vi "NI 5772 (AC) - Digitizer_vDirectDataSend (FPGA).vi"() -> ()   [LabVIEW 2020]
doc: "Example Description:\nThis example demonstrates how to enable Time Interleaved Sampling with the NI 5772 adapter module to achieve a sampling rate of 1.6GS/s. This example continuously acquires records of analog input data from the NI 5772 adapter module. It allows you to select an AI channel, trigger type, and record size. This VI must be compiled before it is run. \n\nRunning the VI:\nThis VI must be run from the NI 5772 - Getting Started (Host).vi. Refer to the host VI documentation for steps regarding running and configuring the FPGA VI. \n\nExecution Steps:\nRefer to the Block Diagram of this VI for execution comments."
uses:
  Controls/AI Trigger Type.ctl
  Controls/Aquire State.ctl
  <vilib>/Platform/TimedLoop/XDataNode/timing_clust.ctl
  <vilib>/Platform/TimedLoop/XDataNode/nitl_modes.ctl
  <vilib>/Platform/TimedLoop/XDataNode/wakeup.ctl
  <vilib>/rvi/Emulation/niFpgaGetClockAttributes.vi
  <vilib>/rvi/Emulation/niFpgaSctlEmulationGetInTimedLoop.vi
  <vilib>/rvi/Emulation/niFpgaEmulationReportErrorSimple.vi
  <vilib>/rvi/eio/common/nirviEmuTemplateMethod_errors.vi
  <vilib>/rvi/Emulation/niFpgaCriticalErrorInLSC.vi
  <vilib>/rvi/Emulation/niFpgaProcessEmulError.vi
  <vilib>/rvi/Emulation/niFpgaEmulationIsFPGAContextNoSignature.vi
  <vilib>/rvi/errors/niFpgaSetErrorForExecOnDevCompSimple.vi
  <vilib>/rvi/eio/common/nirviEmuReportErrorAndStop.vi
  <vilib>/rvi/DataTransferAndStorage/Container/Common/niFpgaContainerGetUniqueNameForEmu.vi
  <vilib>/rvi/FIFO/Fifo_Resource/nirvififoEmulationSetSize.vi
  <vilib>/rvi/FIFO/Fifo_Resource/nirviFifoEmulationQueueMgr.vi
  <instcachedir>/0/nirviFifoEmulationQueueMgr_E5CAEC123FF24DC58D834DCA3CDAA9B5.lvgen/nirviFifoEmulationQueueMgr_E5CAEC123FF24DC58D834DCA3CDAA9B5_004.vi
  <vilib>/Utility/error.llb/Clear Errors.vi
  <vilib>/rvi/FIFO/Fifo_Resource/nirvififoEmulationCreateLock.vi
  <vilib>/rvi/FIFO/Fifo_Resource/nirvififoEmulationObtainLock.vi
  <vilib>/rvi/FIFO/Fifo_Resource/nirvififoEmulationReleaseLock.vi
  <vilib>/rvi/occurrence/nirviWaitOnOccurrenceBase.vi
  <vilib>/rvi/errors/nirviReportUnexpectedCaseInternalError.vi
  <vilib>/rvi/errors/nirviReportUnexpectedCaseInternalError (U32).vi
  <instcachedir>/0/nirviFifoEmulationQueueMgr_E5CAEC123FF24DC58D834DCA3CDAA9B5.lvgen/nirviFifoEmulationQueueMgr_E5CAEC123FF24DC58D834DCA3CDAA9B5_000.vi
  <vilib>/rvi/interface/RandomDataEmulation/niFpgaRandomDataHandleErrors.vi
  <vilib>/rvi/FIFO/Fifo_Resource/nirvififoEmulationDetermineInputValidOut.vi
  <instrlib>/_niInstr/Basic Elements/v1/FPGA/Private/Count Up U64.vi
  <vilib>/eio/EIONode/EIONode.xnode
  <vilib>/rvi/DataTransferAndStorage/Container/XNode/niFpgaContainer.xnode
  <vilib>/rvi/FIFO/Fifo_Resource/nirvififoEmulationRead.vi
  <vilib>/Platform/TimedLoop/XDataNode/XDataNode.xnode
  <vilib>/rvi/interface/RandomDataEmulation/nirviRandomDataFpgaReadWriteTemplate.vi
  <vilib>/rvi/FIFO/Fifo_Resource/nirvififoEmulationWrite.vi
  <vilib>/Platform/TimedLoop/XDataNode/XDNodeRunTimeDep.lvlib
  <instrlib>/_niInstr/Basic Elements/v1/FPGA/niInstr Basic Elements v1 FPGA.lvlib
  Controls/DigitizerState.ctl
  <vilib>/rvi/FIFO/Fifo_Resource/nirvififoEmulationGetNumberOfElementsToRead.vi
  <vilib>/rvi/Memory/Memory_Emulation/nirvimemoryFastEmulation.vi
  <vilib>/rvi/Memory/Memory_Emulation/nirvimemoryEmulation.vi
panel:
  out "DMA FIFO Overflow? 3":bool caption="FIFO Overflow?"
  out "DMA FIFO Overflow? 2":bool caption="FIFO Overflow?"
  out "WaitForWave\nCompletion":u16
  in  "Wave Sampling Rate":sgl
  in  "WaveSampleCount":sgl format="%#_13g"
  in  "Delay (us)":sgl
  in  "AvgCount_powerOf2":i16=1
  out "DMA FIFO Overflow?":bool caption="FIFO Overflow?"
  out "Removed\nElement":u64
  out "AvgCount":u16=1
  in  "vi/nGenTrig":bool
  in  "TrigIn Simulate":bool
  out "Trig Count":u64
  in  "Clear Count":bool
  out "Delay after Trig [cycles]":u16
  out "TS FIFO In Overflow?":bool caption="FIFO Overflow?"
  in  "Samples Per Trigger":u16=512 min=1 step=1
  in  "Arm Trigger":bool
  in  "User Command Commit":bool
  in  "User Command":u8
  out "User Command Idle":bool
  out "User Command Status":u8
  in  "User Data 0":u16
  in  "User Data 1":u8
  out "PLL Locked":bool
  out "User Error":bool
  out "Configured?":bool
  in  "Trigger Level":i16
  in  "Trigger Type":T1
  # "Resource Configuration"
  # "Analog Input"
  # "Clock Configuration"
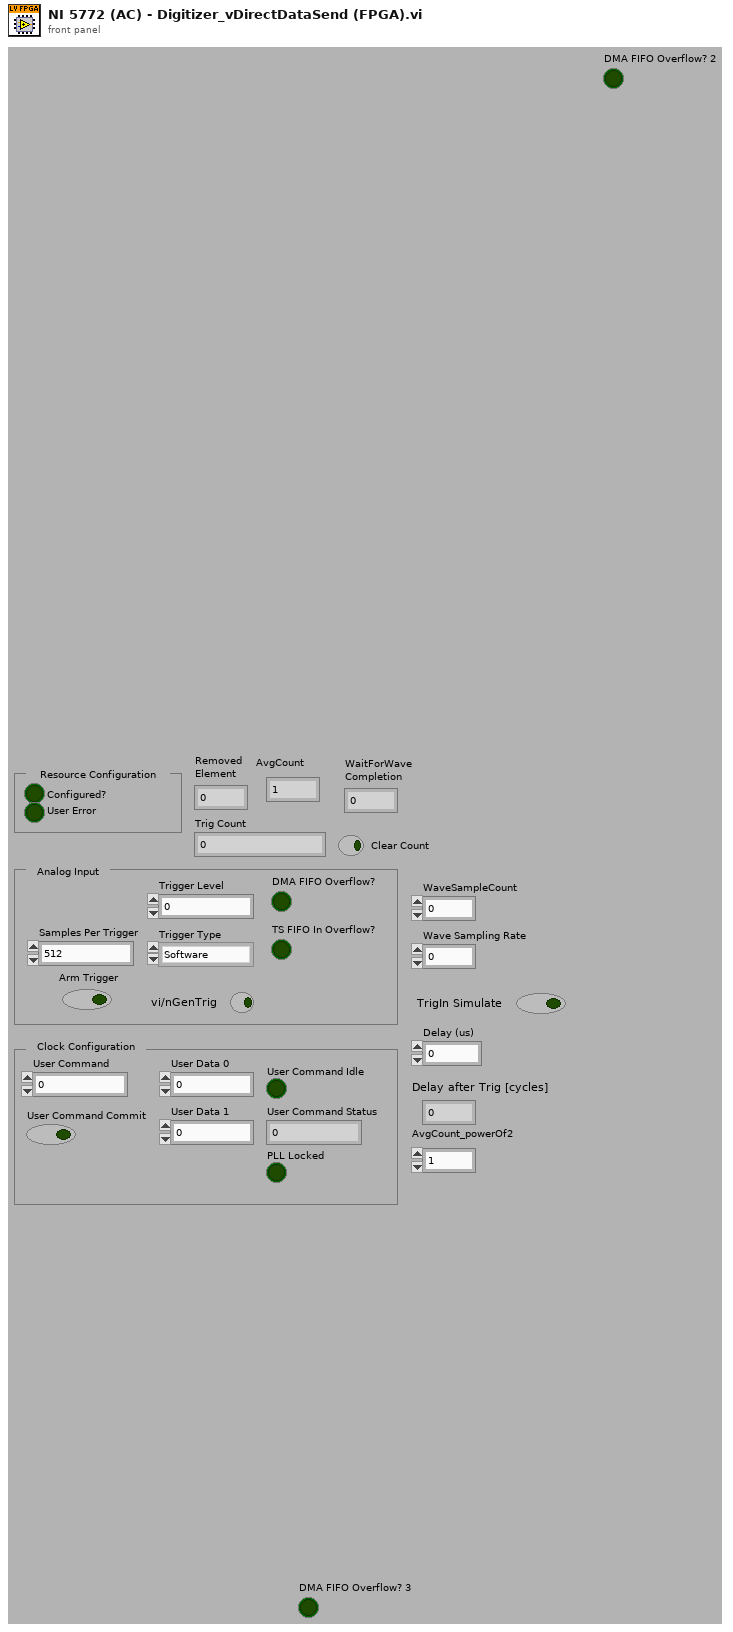
[diagram p1: front panel]
types:
  T1 = typedef "AI Trigger Type.ctl" = enum8{"Software", "Data Edge"}
  T2 = typedef "Aquire State.ctl" = enum8{"Idle", "Wait for Trigger", "AlignWave", "Hold Aquire", "Acquire", "WaitForWaveCompletion", "CheckAvg"}
  T3 = typedef "DigitizerState.ctl" = enum16{"Init", "Build/Clear Accumulator", "GetData", "AverageCountCheck", "SendtoHost"}
  T4 = typedef "XDNodeRunTimeDep.lvlib/timing_clust.ctl" = cluster{"Expected End [f-1]":u64, "Actual End [f-1]":u64, "Finished Late? [f-1]":bool, "Expected End [i-1]":u64, "Actual End [i-1]":u64, "Finished Late? [i-1]":bool, "Expected Start [i]":u64, "Actual Start [i]":u64, "Expected Start [f]":u64, "Actual Start [f]":u64, "Source Name":string, "Structure Name":string, "Period":i64, "Deadline":i64, "Offset":i64, "Start":i64, "Priority":i32, "Timeout":i32, "Mode":T5, "Wakeup Reason":T6, "Error":errorcluster, "Source Type":string, "Secondary Source Type":string, "Global End Time":u64, "Global Start Time":u64, "Frame Duration":u64, "Iteration Duration":u64, "Assigned CPU":i32, "I/O Scan Engine Mode":u32}
  T5 = typedef "XDNodeRunTimeDep.lvlib/nitl_modes.ctl" = enum32{"No Change", "Process missed periods, maintain original phase", "Discard missed periods, maintain original phase", "Process missed periods, ignore original phase", "Discard missed periods, ignore original phase"}
  T6 = typedef "XDNodeRunTimeDep.lvlib/wakeup.ctl" = enum32{"Normal", "Aborted", "Asynchronous wakeup", "Timing source error", "Timed loop error", "Timeout"}
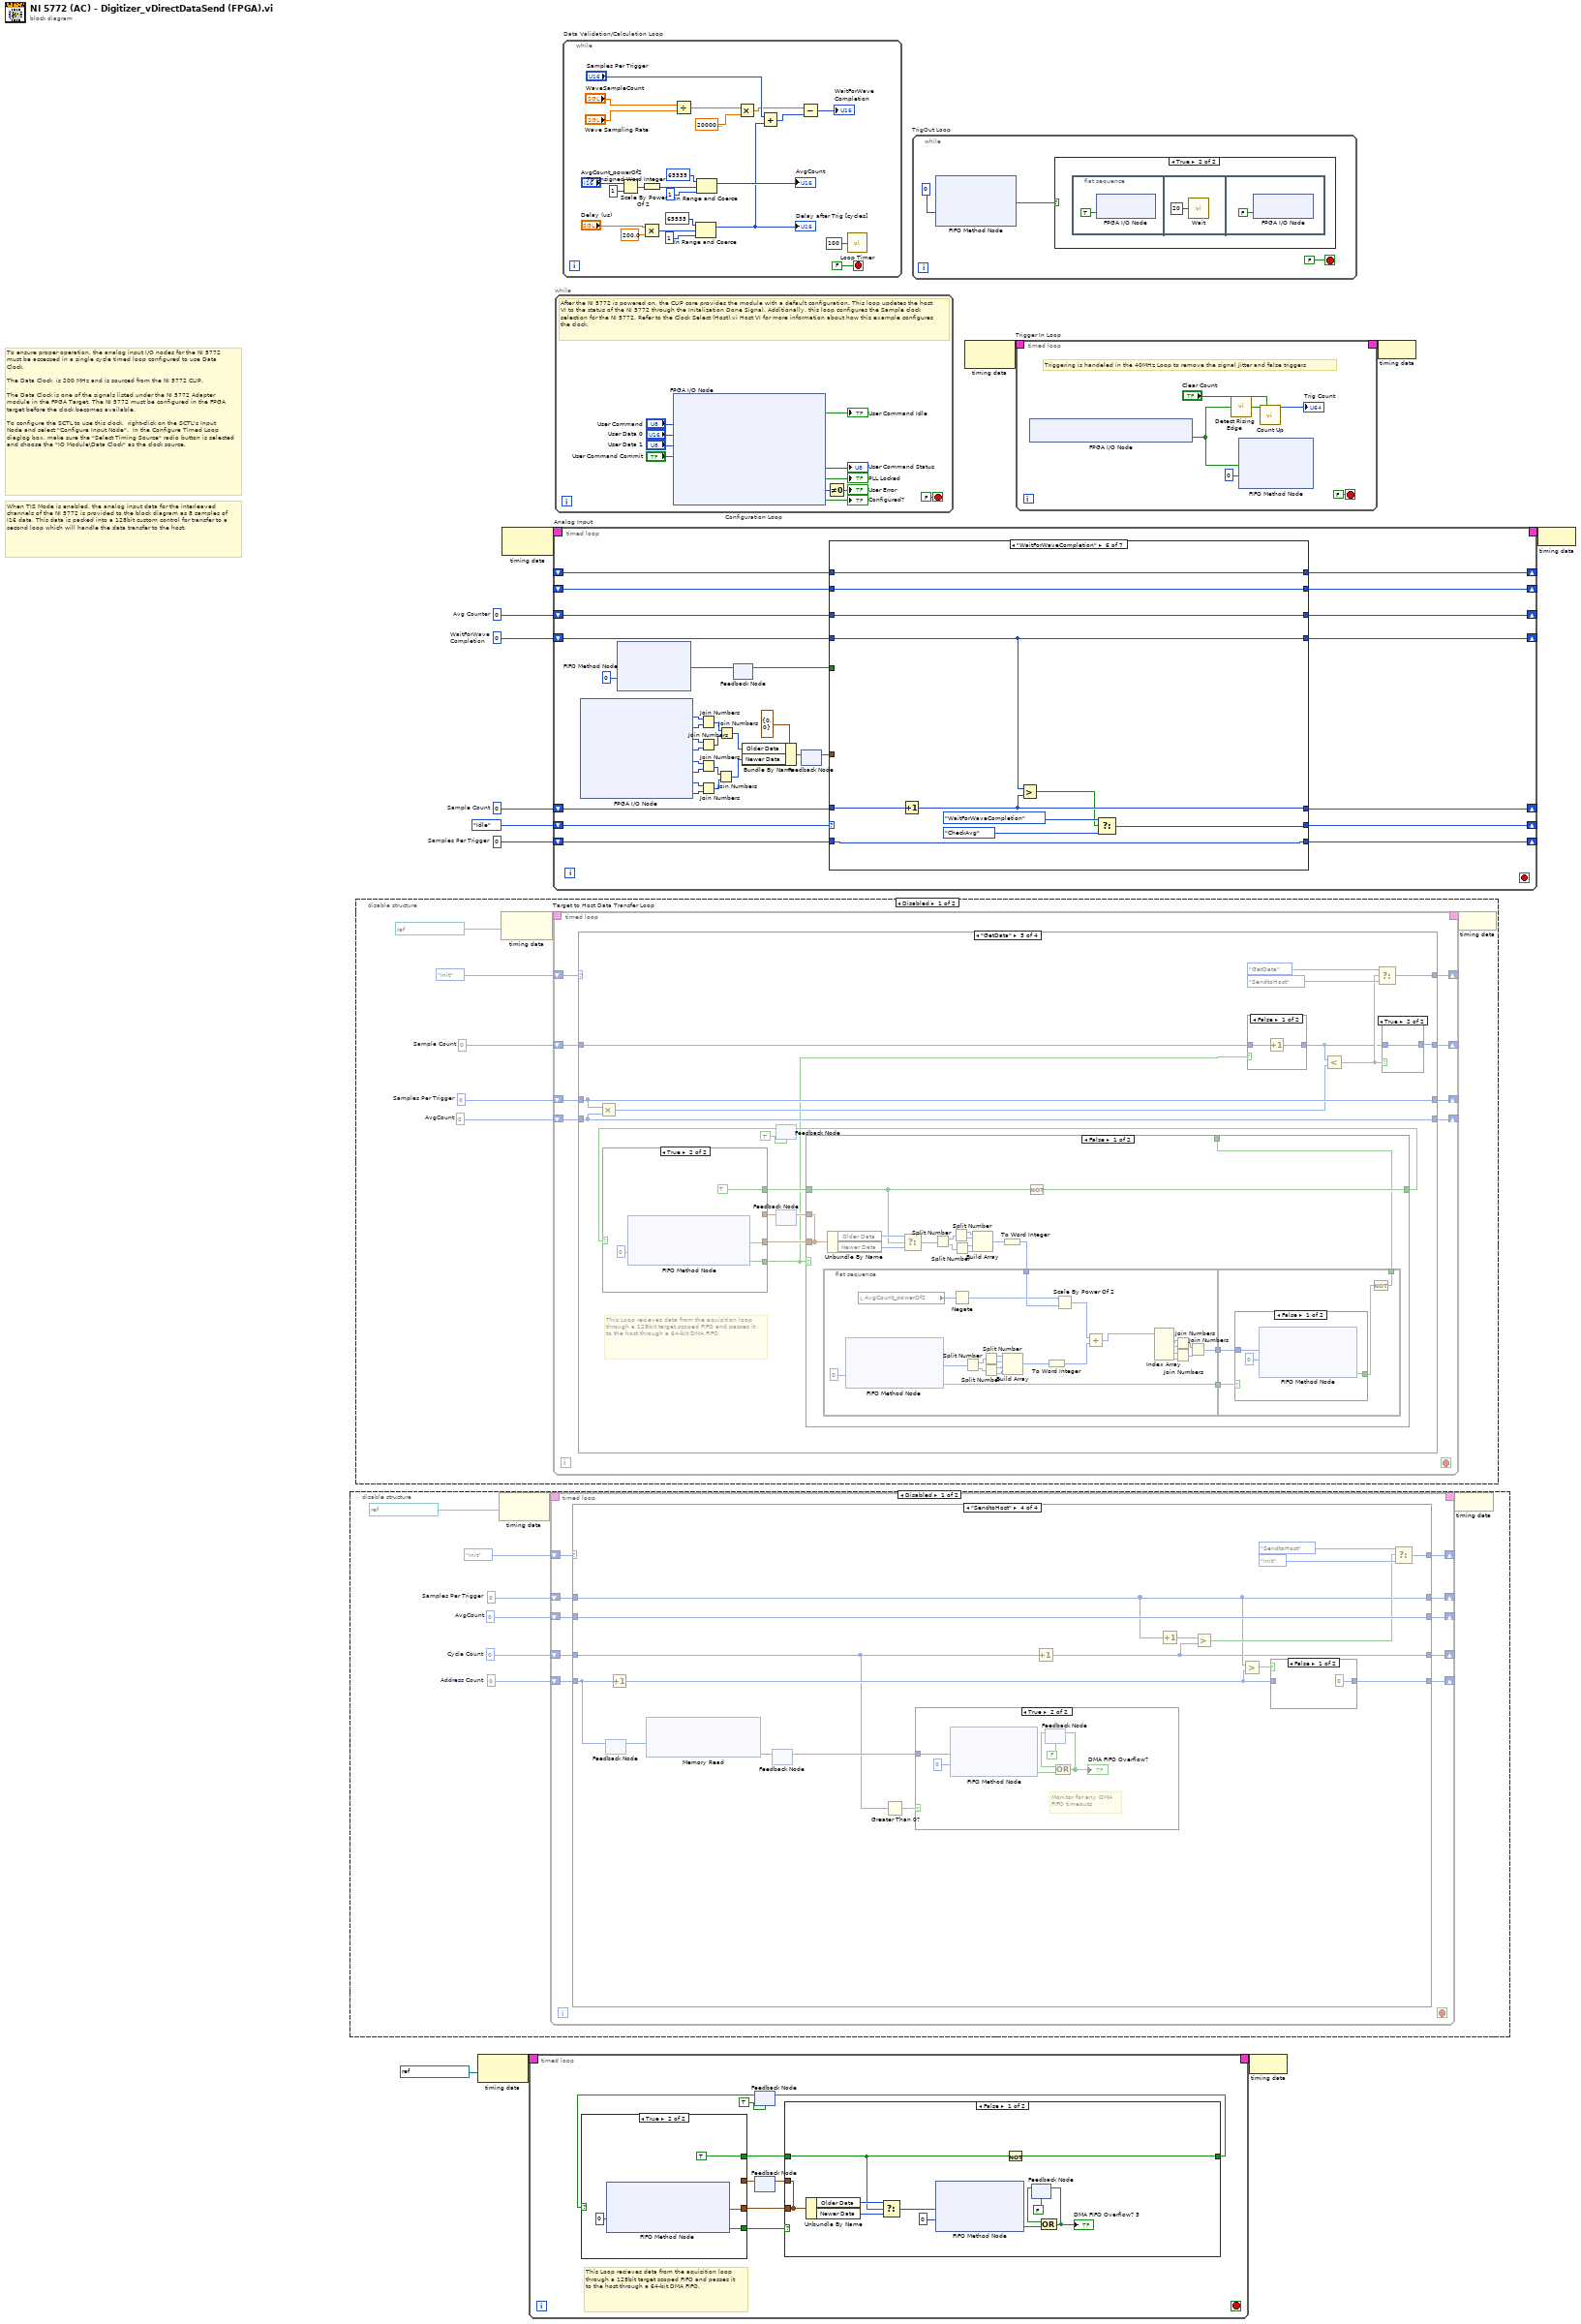
[diagram p0: block diagram]
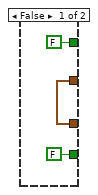
[diagram p2: hidden frame]
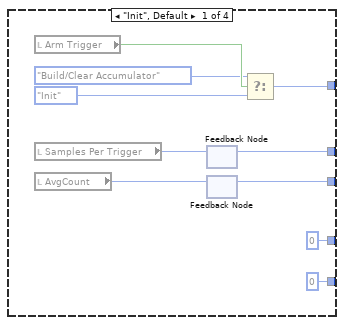
[diagram p4: hidden frame]
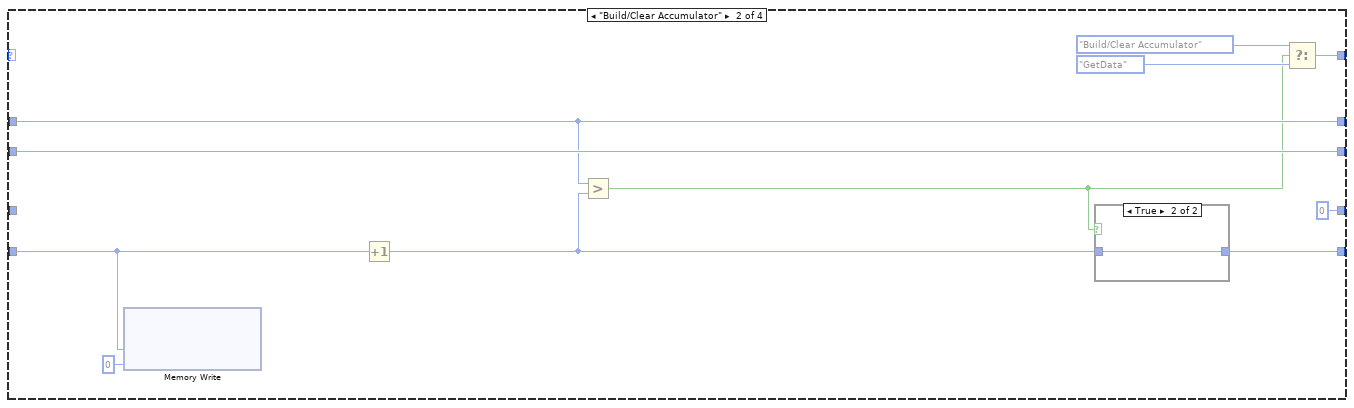
[diagram p5: hidden frame]
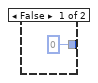
[diagram p6: hidden frame]
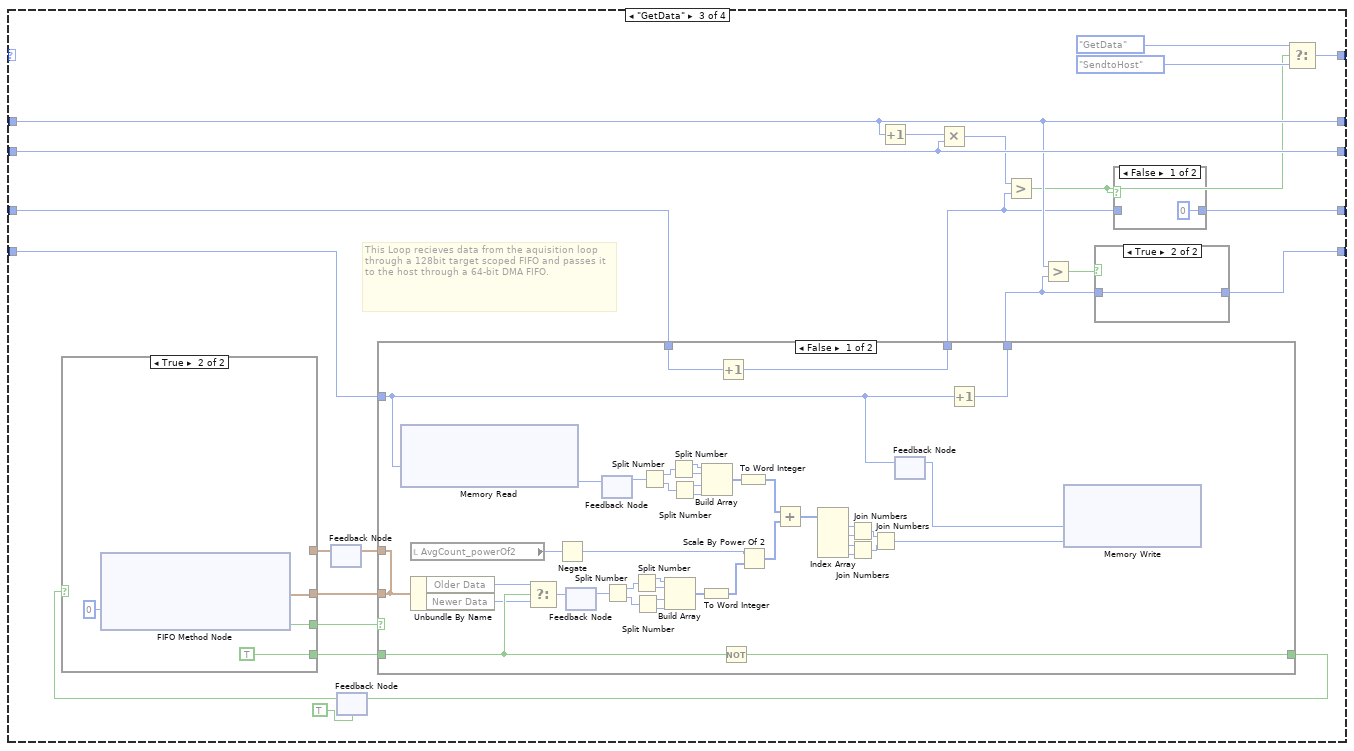
[diagram p7: hidden frame]
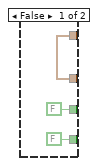
[diagram p9: hidden frame]
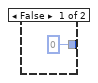
[diagram p11: hidden frame]
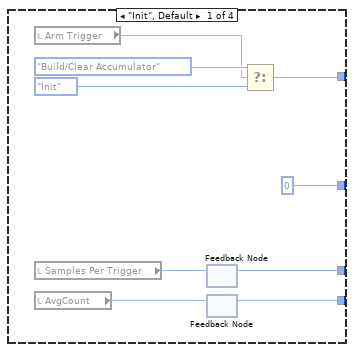
[diagram p15: hidden frame]
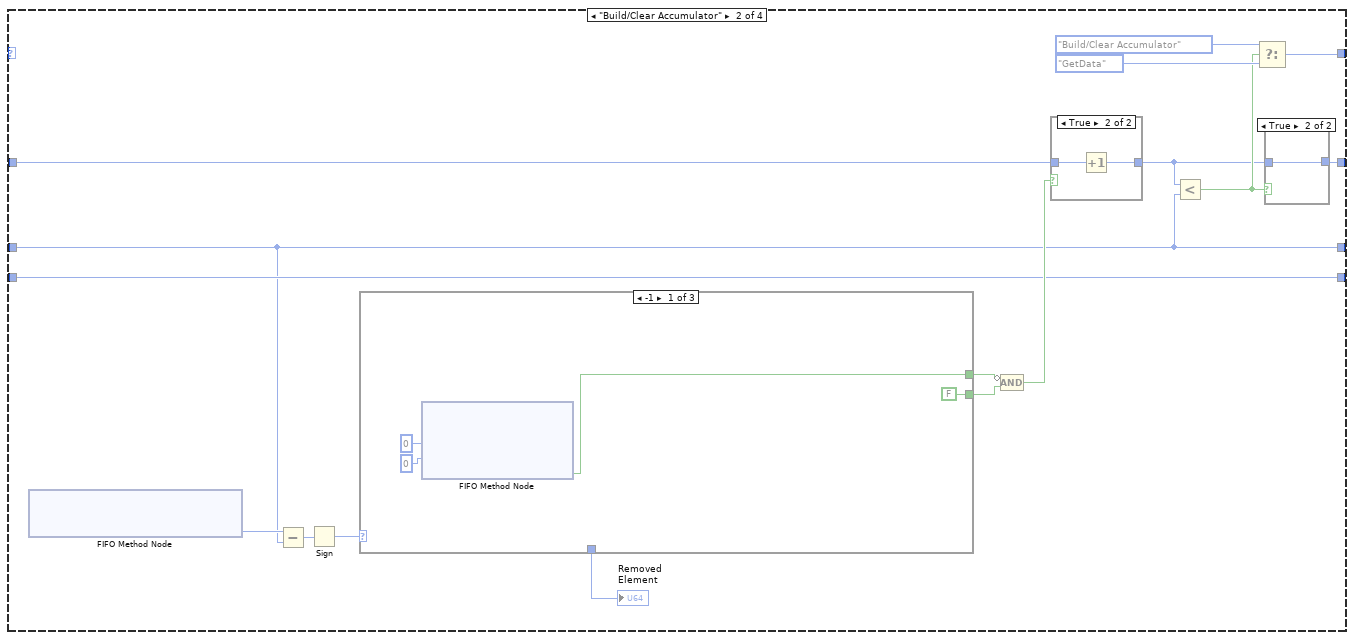
[diagram p16: hidden frame]
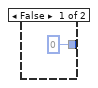
[diagram p17: hidden frame]
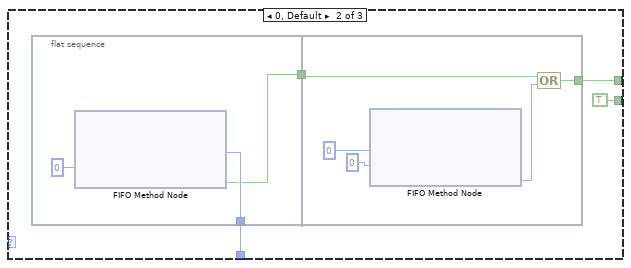
[diagram p19: hidden frame]
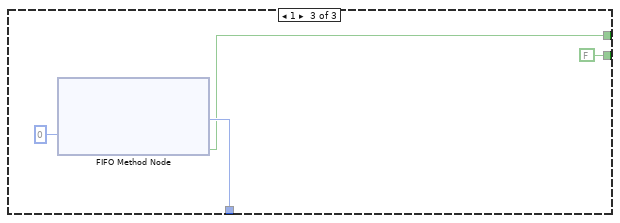
[diagram p20: hidden frame]
diagram:
  w4 = u16 0  # WaitForWave Completion
  w5 = u16 0  # Avg Counter
  w8 = u16 0  # Samples Per Trigger
  w9 = u16 0  # Sample Count
  # "When TIS Mode is enabled, the analog input data for the interleaved channels of the NI 5772 is provided to the block diagram as 8 samples of I16 data. This data is packed into a 128bit custom control for transfer to a second loop which will handle the data transfer to the host."
  # "To ensure proper operation, the analog input I/O nodes for the NI 5772 must be accessed in a single cycle timed loop configured to use Data Clock. \n\nThe Data Clock  is 200 MHz and is sourced from the NI 5772 CLIP.\n\nThe Data Clock is one of the signals listed under the NI 5772 Adapter module in the FPGA Target. The NI 5772 must be configured in the FPGA target before the clock becomes available. \n\nTo configure the SCTL to use this clock,  right-click on the SCTL's Input Node and select \"Configure Input Node\".  In the Configure Timed Loop diaglog box, make sure the \"Select Timing Source\" radio button is selected and choose the \"IO Module\\Data Clock\" as the clock source."
  n1 = disable-structure shown="Disabled" {
    frame Disabled {
      w13 = u32 0  # Cycle Count
      w14 = u32 0  # Address Count
      w15 = u16 0  # AvgCount
      w16 = u16 0  # Samples Per Trigger
      n2 = node-c288(refnum<k21> "100 MHz Clock" ("Source Name")) -> (w20:T4)
      n3 = timed-loop {
        timing: w20 -> [_]
        timing-out: [_] -> w19
        shift-right: [w29] -> _
        shift-left: DigitizerState."Init" -> [w30]
        shift-right: [w28] -> _
        shift-left: w16 -> [w26]
        shift-right: [w27] -> _
        shift-left: w15 -> [w25]
        shift-right: [w23] -> _
        shift-left: w14 -> [w24]
        shift-right: [w21] -> _
        shift-left: w13 -> [w22]
        stop <- _ stop-if-true
        n4 = case shown="\"SendtoHost\"" w30 {
          tunnel: [w35 w45 w74 w146] -> w29
          tunnel: [w34 w48 w58 w136] -> w28
          tunnel: [w33 w49 w64 w149] -> w27
          tunnel: w26 -> [_ w48 w58 w136]
          tunnel: w25 -> [_ w49 w64 w149]
          tunnel: w24 -> [_ w51 w61 w138]
          tunnel: [u32 0 w42 w73 w144] -> w23
          tunnel: w22 -> [_ _ w57 w133]
          tunnel: [u32 0 ("Cycle Count") u32 0 ("Cycle Count") w54 w134] -> w21
          frame "Init", Default {
            n5 = local read "Arm Trigger"() -> (w40:bool)
            n6 = local read "Samples Per Trigger"() -> (w36:u16)
            n7 = local read "AvgCount"() -> (w37:u16)
            n8 = feedback #1() -> (w34:u16)  [unwired: 1 in]
            n9 = feedback-in #1(w36) -> ()
            n10 = feedback #2() -> (w33:u16)  [unwired: 1 in]
            n11 = feedback-in #2(w37) -> ()
            n12 = Select(t=DigitizerState."Build/Clear Accumulator", s=w40, f=DigitizerState."Init") -> (s? t:f=w35:T3)
          }
          frame "Build/Clear Accumulator" {
            n13 = xnode ("Memory Write")("Address"=w51, "Data"=u64 0) -> ()  [unwired: 1 in, 1 out]
            n14 = Increment(x=w51) -> (x+1=w43:u32)
            n15 = Greater?(x=w48, y=w43) -> (0:w44:bool)
            n16 = case shown="True" w44 {
              tunnel: w43 -> [_ w53]
              tunnel: [u32 0 w53] -> w42
              frame False {
              }
              frame True {
              }
            }
            n17 = Select(t=DigitizerState."Build/Clear Accumulator", s=w44, f=DigitizerState."GetData") -> (s? t:f=w45:T3)
          }
          frame "GetData" {
            # "This Loop recieves data from the aquisition loop through a 128bit target scoped FIFO and passes it to the host through a 64-bit DMA FIFO."
            n18 = feedback #3() -> (w68:cluster{"Older Data":u64, "Newer Data":u64})  [unwired: 1 in]
            n19 = feedback #4(TRUE ("Timed Out?")) -> (w67:bool)
            n20 = case shown="True" w67 {
              tunnel: [w79 w82] -> w70
              tunnel: [FALSE ("Timed Out?") w83] -> w72
              tunnel: [FALSE ("Timed Out?") TRUE ("Timed Out?")] -> w71
              tunnel: w68 -> [w79 _]
              frame False {
              }
              frame True {
                n21 = xnode ("FIFO Method Node")("Timeout"=0) -> ("Element"=w82:cluster{"Older Data":u64, "Newer Data":u64}, "Timed Out?"=w83:bool)  [unwired: 1 in, 1 out]
              }
            }
            n22 = case shown="False" w72 {
              tunnel: [w124 w130] -> w66
              tunnel: w71 -> [w125 w130]
              tunnel: w70 -> [w123 w129]
              tunnel: [w123 w129] -> w69
              tunnel: w61 -> [w100 w128]
              tunnel: [w113 w128] -> w60
              tunnel: w57 -> [w89 w127]
              tunnel: [w88 w127] -> w55
              frame False {
                n23 = xnode ("Memory Read")("Address"=w100) -> ("Data"=w91:u64)  [unwired: 1 in, 1 out]
                n24 = local read "AvgCount_powerOf2"() -> (w104:i16)
                n25 = Unbundle By Name(w123) -> ("Older Data"=w126:u64, "Newer Data"=w122:u64)
                n26 = Select(t=w126, s=w125, f=w122) -> (s? t:f=w114:u64)
                n27 = Negate(x=w104) -> (-x=w105:i16)
                n28 = feedback-in #5(w114) -> ()
                n29 = feedback #5() -> (w87:u64)  [unwired: 1 in]
                n30 = feedback-in #6(w91) -> ()
                n31 = feedback #6() -> (w90:u64)  [unwired: 1 in]
                n32 = Split Number(x=w87) -> (hi(x)=w116:u32, lo(x)=w117:u32)
                n33 = Split Number(x=w116) -> (hi(x)=w118:u16, lo(x)=w119:u16)
                n34 = Split Number(x=w117) -> (hi(x)=w120:u16, lo(x)=w121:u16)
                n35 = Split Number(x=w90) -> (hi(x)=w112:u32, lo(x)=w111:u32)
                n36 = Build Array(w118, w119, w120, w121) -> (w115:u16[])
                n37 = Split Number(x=w112) -> (hi(x)=w110:u16, lo(x)=w109:u16)
                n38 = Split Number(x=w111) -> (hi(x)=w108:u16, lo(x)=w107:u16)
                n39 = To Word Integer(number=w115) -> (16bit integer=w103:i16[])
                n40 = Build Array(w110, w109, w108, w107) -> (w106:u16[])
                n41 = Increment(x=w89) -> (x+1=w88:u32)
                n42 = Not(x=w125) -> (.not. x?=w124:bool)
                n43 = To Word Integer(number=w106) -> (16bit integer=w101:i16[])
                n44 = Scale By Power Of 2(n=w105, x=w103) -> (x*2^n=w102:i16[])
                n45 = Add(x=w101, y=w102) -> (x+y=w93:i16[])
                n46 = Index Array(array=w93) -> (element #1=w96:i16, element #2=w97:i16, element #3=w98:i16, element #4=w99:i16)  [unwired: 4 in]
                n47 = Join Numbers(hi=w96, lo=w97) -> ((hi.lo)=w94:u32)
                n48 = Join Numbers(hi=w98, lo=w99) -> ((hi.lo)=w95:u32)
                n49 = Join Numbers(hi=w94, lo=w95) -> ((hi.lo)=w92:u64)
                n50 = feedback-in #7(w100) -> ()
                n51 = feedback #7() -> (w86:u32)  [unwired: 1 in]
                n52 = Increment(x=w100) -> (x+1=w113:u32)
                n53 = xnode ("Memory Write")("Address"=w86, "Data"=w92) -> ()  [unwired: 1 in, 1 out]
              }
              frame True {
              }
            }
            n54 = feedback-in #3(w69) -> ()
            n55 = feedback-in #4(w66) -> ()
            n56 = Increment(x=w58) -> (x+1=w59:u16)
            n57 = Multiply(x=w59, y=w64) -> (x*y=w63:u16)
            n58 = Greater?(x=w63, y=w55) -> (0:w56:bool)
            n59 = Greater?(x=w58, y=w60) -> (0:w62:bool)
            n60 = case shown="True" w62 {
              tunnel: w60 -> [_ w132]
              tunnel: [u32 0 w132] -> w73
              frame False {
              }
              frame True {
              }
            }
            n61 = case shown="False" w56 {
              tunnel: w55 -> [_ w78]
              tunnel: [u32 0 ("Cycle Count") w78] -> w54
              frame False {
              }
              frame True {
              }
            }
            n62 = Select(t=DigitizerState."GetData", s=w56, f=DigitizerState."SendtoHost") -> (s? t:f=w74:T3)
          }
          frame "SendtoHost" {
            n63 = feedback-in #8(w138) -> ()
            n64 = feedback #8() -> (w140:u32)  [unwired: 1 in]
            n65 = Increment(x=w138) -> (x+1=w135:u32)
            n66 = xnode ("Memory Read")("Address"=w140) -> ("Data"=w143:u64)  [unwired: 1 in, 1 out]
            n67 = feedback-in #9(w143) -> ()
            n68 = feedback #9() -> (w142:u64)  [unwired: 1 in]
            n69 = Greater Than 0?(x=w133) -> (x > 0?=w139:bool)
            n70 = case shown="True" w139 {
              tunnel: w142 -> [_ w150]
              frame False {
              }
              frame True {
                # "Monitor for any DMA FIFO timeouts"
                n71 = xnode ("FIFO Method Node")("Element"=w150, "Timeout"=0) -> ("Timed Out?"=w154:bool)  [unwired: 1 in, 1 out]
                n72 = feedback #10(FALSE) -> (w153:bool)
                n73 = Compound Arithmetic op=OR(w153, w154) -> (w155:bool)
                "DMA FIFO Overflow?" <- w155
                n74 = feedback-in #10(w155) -> ()
              }
            }
            n75 = Increment(x=w133) -> (x+1=w134:u32)
            n76 = Increment(x=w136) -> (x+1=w141:u16)
            n77 = Greater?(x=w141, y=w134) -> (0:w145:bool)
            n78 = Greater?(x=w136, y=w135) -> (0:w137:bool)
            n79 = case shown="False" w137 {
              tunnel: w135 -> [_ w157]
              tunnel: [u32 0 w157] -> w144
              frame False {
              }
              frame True {
              }
            }
            n80 = Select(t=DigitizerState."SendtoHost", s=w145, f=DigitizerState."Init") -> (s? t:f=w146:T3)
          }
        }
      }
      n81 = node-c288(w19) -> ()
    }
    frame Enabled {
    }
  }
  n82 = disable-structure shown="Disabled" {
    frame Disabled {
      w164 = u16 0  # Sample Count
      w165 = u16 0  # Samples Per Trigger
      w166 = u16 0  # AvgCount
      n83 = node-c288(refnum<k21> "100 MHz Clock" ("Source Name")) -> (w170:T4)
      n84 = timed-loop "Target to Host Data Transfer Loop" {
        timing: w170 -> [_]
        timing-out: [_] -> w169
        shift-right: [w173] -> _
        shift-left: DigitizerState."Init" -> [w178]
        shift-right: [w177] -> _
        shift-left: w165 -> [w176]
        shift-right: [w175] -> _
        shift-left: w166 -> [w174]
        shift-right: [w171] -> _
        shift-left: w164 -> [w172]
        stop <- _ stop-if-true
        n85 = case shown="\"GetData\"" w178 {
          tunnel: [w186 w191 w239 w313] -> w177
          tunnel: w176 -> [_ w191 w239 w313]
          tunnel: [w184 w192 w238 w320] -> w175
          tunnel: w174 -> [_ w192 w238 w320]
          tunnel: [w180 w199 w233 w316] -> w173
          tunnel: w172 -> [_ w194 w232 w314]
          tunnel: [u16 0 ("Sample Count") w188 w231 w311] -> w171
          frame "Init", Default {
            n86 = local read "Arm Trigger"() -> (w181:bool)
            n87 = local read "Samples Per Trigger"() -> (w187:u16)
            n88 = local read "AvgCount"() -> (w185:u16)
            n89 = feedback #11() -> (w186:u16)  [unwired: 1 in]
            n90 = feedback-in #11(w187) -> ()
            n91 = feedback #12() -> (w184:u16)  [unwired: 1 in]
            n92 = feedback-in #12(w185) -> ()
            n93 = Select(t=DigitizerState."Build/Clear Accumulator", s=w181, f=DigitizerState."Init") -> (s? t:f=w180:T3)
          }
          frame "Build/Clear Accumulator" {
            n94 = xnode ("FIFO Method Node")() -> ("Number of Elements to Read"=w203:u32)  [unwired: 1 in, 1 out]
            n95 = Subtract(x=w203, y=w191) -> (x-y=w202:i8)
            n96 = Sign(1:w202) -> (0:w201:i8)
            n97 = case shown="-1" w201 {
              tunnel: [_ w216 w227] -> w200
              tunnel: [w210 w214 w226] -> w196
              tunnel: [FALSE TRUE FALSE] -> w195
              frame -1 {
                n98 = xnode ("FIFO Method Node")("Element"=u64 0, "Timeout"=0) -> ("Timed Out?"=w210:bool)  [unwired: 1 in, 1 out]
              }
              frame 0, Default {
                n99 = flat-sequence {
                  tunnel: [w218] -> w216
                  tunnel: [w217] -> w215
                  tunnel: w215 -> [w222]
                  tunnel: [w220] -> w214
                  frame #0 {
                    n100 = xnode ("FIFO Method Node")("Timeout"=0) -> ("Element"=w218:u64, "Timed Out?"=w217:bool)  [unwired: 1 in, 1 out]
                  }
                  frame #1 {
                    n101 = xnode ("FIFO Method Node")("Element"=u64 0 ("y"), "Timeout"=0) -> ("Timed Out?"=w221:bool)  [unwired: 1 in, 1 out]
                    n102 = Compound Arithmetic op=OR(w222, w221) -> (w220:bool)
                  }
                }
              }
              frame 1 {
                n103 = xnode ("FIFO Method Node")("Timeout"=0) -> ("Element"=w227:u64, "Timed Out?"=w226:bool)  [unwired: 1 in, 1 out]
              }
            }
            "Removed\nElement" <- w200
            n104 = Compound Arithmetic op=AND(invert w196, w195) -> (w193:bool)
            n105 = case shown="True" w193 {
              tunnel: w194 -> [w206 w208]
              tunnel: [w206 w207] -> w189
              frame False {
              }
              frame True {
                n106 = Increment(x=w208) -> (x+1=w207:u16)
              }
            }
            n107 = Less?(x=w189, y=w191) -> (x < y?=w190:bool)
            n108 = Select(t=DigitizerState."Build/Clear Accumulator", s=w190, f=DigitizerState."GetData") -> (s? t:f=w199:T3)
            n109 = case shown="True" w190 {
              tunnel: [u16 0 ("Sample Count") w205] -> w188
              tunnel: w189 -> [_ w205]
              frame False {
              }
              frame True {
              }
            }
          }
          frame "GetData" {
            # "This Loop recieves data from the aquisition loop through a 128bit target scoped FIFO and passes it to the host through a 64-bit DMA FIFO."
            n110 = Multiply(x=w239, y=w238) -> (x*y=w230:u16)
            n111 = feedback #13(TRUE ("Timed Out?")) -> (w244:bool)
            n112 = feedback #14() -> (w243:cluster{"Older Data":u64, "Newer Data":u64})  [unwired: 1 in]
            n113 = case shown="True" w244 {
              tunnel: [w252 w255] -> w241
              tunnel: [FALSE ("Timed Out?") w256] -> w229
              tunnel: [FALSE ("Timed Out?") TRUE ("Timed Out?")] -> w240
              tunnel: w243 -> [w252 _]
              frame False {
              }
              frame True {
                n114 = xnode ("FIFO Method Node")("Timeout"=0) -> ("Element"=w255:cluster{"Older Data":u64, "Newer Data":u64}, "Timed Out?"=w256:bool)  [unwired: 1 in, 1 out]
              }
            }
            n115 = case shown="False" w229 {
              tunnel: [w273 w309] -> w245
              tunnel: w240 -> [w274 w309]
              tunnel: w241 -> [w272 w308]
              tunnel: [w272 w308] -> w242
              tunnel: [w260 FALSE ("increment")] -> _
              frame False {
                n116 = flat-sequence {
                  tunnel: [w276] -> w264
                  tunnel: [w287] -> w262
                  tunnel: w259 -> [w283]
                  tunnel: w264 -> [w302]
                  tunnel: [w299] -> w260
                  tunnel: w262 -> [w301]
                  frame #0 {
                    n117 = xnode ("FIFO Method Node")("Timeout"=0) -> ("Element"=w286:u64, "Timed Out?"=w287:bool)  [unwired: 1 in, 1 out]
                    n118 = local read "AvgCount_powerOf2"() -> (w285:i16)
                    n119 = Negate(x=w285) -> (-x=w284:i16)
                    n120 = Split Number(x=w286) -> (hi(x)=w292:u32, lo(x)=w293:u32)
                    n121 = Split Number(x=w292) -> (hi(x)=w294:u16, lo(x)=w295:u16)
                    n122 = Split Number(x=w293) -> (hi(x)=w296:u16, lo(x)=w297:u16)
                    n123 = Build Array(w294, w295, w296, w297) -> (w298:u16[])
                    n124 = To Word Integer(number=w298) -> (16bit integer=w290:i16[])
                    n125 = Scale By Power Of 2(n=w284, x=w283) -> (x*2^n=w282:i16[])
                    n126 = Add(x=w282, y=w290) -> (x+y=w281:i16[])
                    n127 = Index Array(array=w281) -> (element #1=w280:i16, element #2=w279:i16, element #3=w278:i16, element #4=w277:i16)  [unwired: 4 in]
                    n128 = Join Numbers(hi=w280, lo=w279) -> ((hi.lo)=w289:u32)
                    n129 = Join Numbers(hi=w278, lo=w277) -> ((hi.lo)=w288:u32)
                    n130 = Join Numbers(hi=w289, lo=w288) -> ((hi.lo)=w276:u64)
                  }
                  frame #1 {
                    n131 = case shown="False" w301 {
                      tunnel: w302 -> [w304 _]
                      tunnel: [w303 TRUE ("Timed Out?")] -> w300
                      frame False {
                        n132 = xnode ("FIFO Method Node")("Element"=w304, "Timeout"=0) -> ("Timed Out?"=w303:bool)  [unwired: 1 in, 1 out]
                      }
                      frame True {
                      }
                    }
                    n133 = Not(x=w300) -> (.not. x?=w299:bool)
                  }
                }
                n134 = Unbundle By Name(w272) -> ("Older Data"=w275:u64, "Newer Data"=w271:u64)
                n135 = Select(t=w275, s=w274, f=w271) -> (s? t:f=w261:u64)
                n136 = Split Number(x=w261) -> (hi(x)=w265:u32, lo(x)=w266:u32)
                n137 = Split Number(x=w265) -> (hi(x)=w267:u16, lo(x)=w268:u16)
                n138 = Split Number(x=w266) -> (hi(x)=w269:u16, lo(x)=w270:u16)
                n139 = Build Array(w267, w268, w269, w270) -> (w263:u16[])
                n140 = To Word Integer(number=w263) -> (16bit integer=w259:i16[])
                n141 = Not(x=w274) -> (.not. x?=w273:bool)
              }
              frame True {
              }
            }
            n142 = feedback-in #13(w245) -> ()
            n143 = feedback-in #14(w242) -> ()
            n144 = case shown="False" w229 {
              tunnel: w232 -> [w250 w251]
              tunnel: [w249 w251] -> w234
              frame False {
                n145 = Increment(x=w250) -> (x+1=w249:u16)
              }
              frame True {
              }
            }
            n146 = Less?(x=w234, y=w230) -> (x < y?=w235:bool)
            n147 = Select(t=DigitizerState."GetData", s=w235, f=DigitizerState."SendtoHost") -> (s? t:f=w233:T3)
            n148 = case shown="True" w235 {
              tunnel: [u16 0 ("Sample Count") w248] -> w231
              tunnel: w234 -> [_ w248]
              frame False {
              }
              frame True {
              }
            }
          }
          frame "SendtoHost" {
            n149 = xnode ("FIFO Method Node")("Timeout"=0) -> ("Element"=w319:u64, "Timed Out?"=w310:bool)  [unwired: 1 in, 1 out]
            n150 = case shown="False" w310 {
              tunnel: w319 -> [w322 _]
              frame False {
                n151 = xnode ("FIFO Method Node")("Element"=w322, "Timeout"=0) -> ("Timed Out?"=w324:bool)  [unwired: 1 in, 1 out]
                n152 = feedback #15(FALSE) -> (w325:bool)
                n153 = Compound Arithmetic op=OR(w325, w324) -> (w323:bool)
                "DMA FIFO Overflow? 2" <- w323
                n154 = feedback-in #15(w323) -> ()
              }
              frame True {
              }
            }
            n155 = Increment(x=w314) -> (x+1=w315:u16)
            n156 = Less?(x=w315, y=w313) -> (x < y?=w312:bool)
            n157 = case shown="False" w312 {
              tunnel: [u16 0 ("Sample Count") w329] -> w311
              tunnel: w315 -> [_ w329]
              frame False {
              }
              frame True {
              }
            }
            n158 = Select(t=DigitizerState."SendtoHost", s=w312, f=DigitizerState."Init") -> (s? t:f=w316:T3)
          }
        }
      }
      n159 = node-c288(w169) -> ()
    }
    frame Enabled {
    }
  }
  n160 = node-c288(refnum<k21> "100 MHz Clock" ("Source Name")) -> (w3:T4)
  n161 = node-c288() -> (w12:T4)  [unwired: 1 in]
  n162 = timed-loop {
    timing: w3 -> [_]
    timing-out: [_] -> w2
    stop <- _ stop-if-true
    # "This Loop recieves data from the aquisition loop through a 128bit target scoped FIFO and passes it to the host through a 64-bit DMA FIFO."
    n163 = feedback #16(TRUE ("Timed Out?")) -> (w338:bool)
    n164 = feedback #17() -> (w339:cluster{"Older Data":u64, "Newer Data":u64})  [unwired: 1 in]
    n165 = case shown="True" w338 {
      tunnel: [w344 w347] -> w341
      tunnel: [FALSE ("Timed Out?") w348] -> w343
      tunnel: [FALSE ("Timed Out?") TRUE ("Timed Out?")] -> w342
      tunnel: w339 -> [w344 _]
      frame False {
      }
      frame True {
        n166 = xnode ("FIFO Method Node")("Timeout"=0) -> ("Element"=w347:cluster{"Older Data":u64, "Newer Data":u64}, "Timed Out?"=w348:bool)  [unwired: 1 in, 1 out]
      }
    }
    n167 = case shown="False" w343 {
      tunnel: [w359 w363] -> w337
      tunnel: w342 -> [w360 w363]
      tunnel: w341 -> [w358 w362]
      tunnel: [w358 w362] -> w340
      frame False {
        n168 = Unbundle By Name(w358) -> ("Older Data"=w361:u64, "Newer Data"=w357:u64)
        n169 = Select(t=w361, s=w360, f=w357) -> (s? t:f=w351:u64)
        n170 = xnode ("FIFO Method Node")("Element"=w351, "Timeout"=0) -> ("Timed Out?"=w353:bool)  [unwired: 1 in, 1 out]
        n171 = Not(x=w360) -> (.not. x?=w359:bool)
        n172 = feedback #18(FALSE) -> (w354:bool)
        n173 = Compound Arithmetic op=OR(w354, w353) -> (w352:bool)
        "DMA FIFO Overflow? 3" <- w352
        n174 = feedback-in #18(w352) -> ()
      }
      frame True {
      }
    }
    n175 = feedback-in #16(w337) -> ()
    n176 = feedback-in #17(w340) -> ()
  }
  n177 = timed-loop "Analog Input" {
    timing: w12 -> [_]
    timing-out: [_] -> w11
    shift-right: [w398] -> _
    shift-left: Aquire_State."Idle" ("Acquire State") -> [w388]
    shift-right: [w399] -> _
    shift-left: w9 -> [w389]
    shift-right: [w397] -> _
    shift-left: w8 -> [w387]
    shift-right: [w374] -> _
    shift-left: _ -> [w373]
    shift-right: [w372] -> _
    shift-left: _ -> [w371]
    shift-right: [w369] -> _
    shift-left: w5 -> [w370]
    shift-right: [w367] -> _
    shift-left: w4 -> [w366]
    stop <- _ stop-if-true
    n178 = xnode "FPGA I/O Node"() -> ("IO Module\\AI 1 Data N-3"=w380:i16, "IO Module\\AI 0 Data N-3"=w379:i16, "IO Module\\AI 1 Data N-2"=w378:i16, "IO Module\\AI 0 Data N-2"=w377:i16, "IO Module\\AI 1 Data N-1"=w381:i16, "IO Module\\AI 0 Data N-1"=w382:i16, "IO Module\\AI 1 Data N"=w383:i16, "IO Module\\AI 0 Data N"=w384:i16)  [unwired: 8 in, 8 out]
    n179 = xnode ("FIFO Method Node")("Timeout"=0) -> ("Element"=w375:bool)  [unwired: 1 in, 2 out]
    n180 = Join Numbers(hi=w380, lo=w379) -> ((hi.lo)=w392:u32)
    n181 = Join Numbers(hi=w378, lo=w377) -> ((hi.lo)=w394:u32)
    n182 = Join Numbers(hi=w381, lo=w382) -> ((hi.lo)=w393:u32)
    n183 = Join Numbers(hi=w383, lo=w384) -> ((hi.lo)=w395:u32)
    n184 = Join Numbers(hi=w393, lo=w395) -> ((hi.lo)=w385:u64)
    n185 = Join Numbers(hi=w392, lo=w394) -> ((hi.lo)=w386:u64)
    n186 = feedback-in #19(w375) -> ()
    n187 = feedback #19() -> (w368:bool)  [unwired: 1 in]
    n188 = Bundle By Name(cluster=cluster{"Older Data":u64, "Newer Data":u64} {"Older Data"=0, "Newer Data"=0} ("Element"), "Older Data"=w386, "Newer Data"=w385) -> (w390:cluster{"Older Data":u64, "Newer Data":u64})
    n189 = feedback #20() -> (w396:cluster{"Older Data":u64, "Newer Data":u64})  [unwired: 1 in]
    n190 = feedback-in #20(w390) -> ()
    n191 = case shown="\"WaitForWaveCompletion\"" w388 {
      tunnel: [u16 0 u16 0 w452 w464 w473 w495 u16 0] -> w399
      tunnel: w389 -> [_ _ w452 w463 w488 w497 _]
      tunnel: [w411 w423 w455 w467 w487 w500 w511] -> w398
      tunnel: [w408 w427 w453 w465 w484 w498 w509] -> w397
      tunnel: w387 -> [_ w427 w453 w465 w484 w498 w509]
      tunnel: w396 -> [_ w426 _ _ w483 _ _]
      tunnel: w368 -> [_ w421 _ _ _ _ _]
      tunnel: [w406 w419 w451 w462 w477 w496 w508] -> w374
      tunnel: w373 -> [_ w419 w451 w462 w477 w496 w508]
      tunnel: [w404 w418 w450 w460 w476 w493 w506] -> w372
      tunnel: w371 -> [_ w418 w450 w460 w476 w493 w506]
      tunnel: [u16 0 ("Avg Count") w417 w449 w459 w475 w492 w505] -> w369
      tunnel: w370 -> [_ w417 w449 w459 w475 w492 w507]
      tunnel: [w400 w415 w447 w457 w471 w491 w502] -> w367
      tunnel: w366 -> [_ w415 w447 w457 w471 w491 w502]
      frame "Idle", Default {
        # "This state will wait for the host VI to arm the trigger."
        n192 = feedback-in #21("Arm Trigger") -> ()
        n193 = feedback #21() -> (w409:bool)  [unwired: 1 in]
        n194 = local read "WaitForWave\nCompletion"() -> (w401:u16)
        n195 = Select(t=Aquire_State."Wait for Trigger" ("Acquire State"), s=w409, f=Aquire_State."Idle" ("Acquire State")) -> (s? t:f=w411:T2)
        n196 = local read "Delay after Trig [cycles]"() -> (w407:u16)
        n197 = local read "AvgCount"() -> (w405:u16)
        n198 = local read "Samples Per Trigger"() -> (w402:u16)
        n199 = feedback #22() -> (w406:u16)  [unwired: 1 in]
        n200 = feedback-in #22(w407) -> ()
        n201 = feedback #23() -> (w404:u16)  [unwired: 1 in]
        n202 = feedback-in #23(w405) -> ()
        n203 = feedback #24() -> (w400:u16)  [unwired: 1 in]
        n204 = feedback-in #24(w401) -> ()
        n205 = feedback-in #25(w402) -> ()
        n206 = feedback #25() -> (w408:u16)  [unwired: 1 in]
      }
      frame "Wait for Trigger" {
        # "After the trigger is armed, this state monitors for the specific trigger condition to begin the acquisition."
        n207 = feedback-in #26("Trigger Type") -> ()
        n208 = feedback #26() -> (w420:T1)  [unwired: 1 in]
        n209 = case shown="\"Software\", Default" w420 {
          tunnel: w426 -> [_ w446]
          tunnel: [w437 w438] -> w416
          tunnel: w421 -> [w432 _]
          frame "Software", Default {
            n210 = Compound Arithmetic op=AND(w432, invert "vi/nGenTrig") -> (w436:bool)
            n211 = Compound Arithmetic op=AND("vi/nGenTrig", "TrigIn Simulate") -> (w434:bool)
            n212 = Compound Arithmetic op=OR(w436, w434) -> (w431:bool)
            n213 = call <instrlib>:"Detect Rising Edge.vi"("signal"=w431) -> ("edge detected"=w437:bool)  [unwired: 14 in]
          }
          frame "Data Edge" {
            # "Begins the acquisition after the analog input rises above the trigger level."
            n214 = Unbundle By Name(w446) -> ("Older Data"=w444:u64, "Newer Data"=w442:u64)
            n215 = feedback-in #27("Trigger Level") -> ()
            n216 = feedback #27() -> (w440:i16)  [unwired: 1 in]
            n217 = feedback-in #28(w444) -> ()
            n218 = feedback #28() -> (w439:u64)  [unwired: 1 in]
            n219 = feedback-in #29(w442) -> ()
            n220 = feedback #29() -> (w441:u64)  [unwired: 1 in]
            n221 = call "Data Edge Trigger 8 Samples.vi"("Trigger Level"=w440, "Newer Data In"=w441, "Older Data In"=w439) -> ("Trigger"=w445:bool)  [unwired: 8 in]
            n222 = feedback-in #30(w445) -> ()
            n223 = feedback #30() -> (w438:bool)  [unwired: 1 in]
          }
        }
        n224 = case shown="True" w416 {
          selector: w416 -> [_ w430]
          frame False {
          }
          frame True {
            n225 = xnode ("FIFO Method Node")("Element"=w430, "Timeout"=0) -> ()  [unwired: 1 in, 2 out]
          }
        }
        n226 = Select(t=Aquire_State."AlignWave" ("Acquire State"), s=w416, f=Aquire_State."Wait for Trigger") -> (s? t:f=w423:T2)
      }
      frame "AlignWave" {
        n227 = xnode "FPGA I/O Node"() -> ("PXI_Trig0"=w448:bool)  [unwired: 1 in, 1 out]
        n228 = Select(t=Aquire_State."Hold Aquire" ("Acquire State"), s=w448, f=Aquire_State."AlignWave" ("Acquire State")) -> (s? t:f=w455:T2)
      }
      frame "Hold Aquire" {
        n229 = Increment(x=w463) -> (x+1=w461:u16)
        n230 = Greater?(x=w462, y=w461) -> (0:w458:bool)
        n231 = Select(t=Aquire_State."Hold Aquire" ("Acquire State"), s=w458, f=Aquire_State."Acquire" ("Acquire State")) -> (s? t:f=w467:T2)
        n232 = case shown="True" w458 {
          tunnel: [u16 0 w470] -> w464
          tunnel: w461 -> [_ w470]
          frame False {
          }
          frame True {
          }
        }
      }
      frame "Acquire" {
        # "Monitor for any  FIFO timeouts"
        # "While in this state, data is pushed into a DMA FIFO until the desired number of samples per record have been acquired."
        n233 = xnode ("FIFO Method Node")("Element"=w483, "Timeout"=0) -> ("Timed Out?"=w478:bool)  [unwired: 1 in, 1 out]
        n234 = Increment(x=w488) -> (x+1=w474:u16)
        n235 = Less?(x=w474, y=w484) -> (x < y?=w472:bool)
        n236 = feedback #31(FALSE) -> (w479:bool)
        n237 = Or(x=w479, y=w478) -> (x .or. y?=w480:bool)
        "TS FIFO In Overflow?" <- w480
        n238 = feedback-in #31(w480) -> ()
        n239 = Select(t=Aquire_State."Acquire" ("Acquire State"), s=w472, f=Aquire_State."WaitForWaveCompletion" ("Acquire State")) -> (s? t:f=w487:T2)
        n240 = case shown="False" w472 {
          tunnel: w474 -> [_ w490]
          tunnel: [u16 0 w490] -> w473
          frame False {
          }
          frame True {
          }
        }
      }
      frame "WaitForWaveCompletion" {
        n241 = Increment(x=w497) -> (x+1=w495:u16)
        n242 = Greater?(x=w491, y=w495) -> (0:w494:bool)
        n243 = Select(t=Aquire_State."WaitForWaveCompletion" ("Acquire State"), s=w494, f=Aquire_State."CheckAvg" ("Acquire State")) -> (s? t:f=w500:T2)
      }
      frame "CheckAvg" {
        n244 = Increment(x=w507) -> (x+1=w505:u16)
        n245 = Greater?(x=w506, y=w505) -> (0:w503:bool)
        n246 = Select(t=Aquire_State."AlignWave" ("Acquire State"), s=w503, f=Aquire_State."Idle") -> (s? t:f=w511:T2)
        n247 = xnode ("FIFO Method Node")("Element"=w503, "Timeout"=0) -> ()  [unwired: 1 in, 2 out]
      }
    }
  }
  n248 = while "Configuration Loop" {
    stop <- FALSE stop-if-true
    # "After the NI 5772 is powered on, the CLIP core provides the module with a default configuration. This loop updates the host VI to the status of the NI 5772 through the Initalization Done Signal. Additionally, this loop configures the Sample clock selection for the NI 5772. Refer to the Clock Select (Host).vi Host VI for more information about how this example configures the clock."
    n249 = xnode "FPGA I/O Node"("IO Module\\User Command"="User Command", "IO Module\\User Data 0"="User Data 0", "IO Module\\User Data 1"="User Data 1", "IO Module\\User Command Commit"="User Command Commit") -> ("IO Module\\User Command Idle"=→"User Command Idle":bool, "IO Module\\User Command Status"=→"User Command Status":u8, "IO Module\\PLL Locked"=→"PLL Locked":bool, "IO Module\\User Error"=w521:u8, "IO Module\\Initialization Done"=→"Configured?":bool)  [unwired: 9 in, 9 out]
    n250 = Not Equal To 0?(x=w521) -> (x != 0?=→"User Error":bool)
  }
  n251 = while "Data Validation/Calculation Loop" {
    stop <- FALSE stop-if-true
    n252 = Scale By Power Of 2(n="AvgCount_powerOf2", x=1 ("Timeout")) -> (x*2^n=w547:i32)
    n253 = To Unsigned Word Integer(number=w547) -> (unsigned 16bit integer=w544:u16)
    n254 = Multiply(x="Delay (us)", y=sgl 200.0) -> (x*y=w540:u16)
    n255 = Divide(x="WaveSampleCount", y="Wave Sampling Rate") -> (x/y=w531:sgl)
    n256 = In Range and Coerce(upper limit=u16 65535, x=w540, lower limit=u16 1) -> (coerced(x)=w532:u16)  [unwired: 1 out]
    "Delay after Trig [cycles]" <- w532
    n257 = In Range and Coerce(upper limit=u16 65535, x=w544, lower limit=u16 1) -> (coerced(x)=→"AvgCount":u16)  [unwired: 1 out]
    n258 = Multiply(x=w531, y=sgl 200000000.0) -> (x*y=w528:sgl)
    n259 = Add(x="Samples Per Trigger", y=w532) -> (x+y=w529:u16)
    n260 = Subtract(x=w528, y=w529) -> (x-y=→"WaitForWave\nCompletion":u16)
    n261 = call "Loop Timer"("Count(uSec)"=u32 100 ("Count(mSec)")) -> ()  [unwired: 1 out]
  }
  n262 = while "TrigOut Loop" {
    stop <- FALSE stop-if-true
    n263 = xnode ("FIFO Method Node")("Timeout"=0) -> ("Element"=w550:bool)  [unwired: 1 in, 2 out]
    n264 = case shown="True" w550 {
      frame False {
      }
      frame True {
        n265 = flat-sequence {
          frame #0 {
            n266 = xnode "FPGA I/O Node"("PXI_Trig1"=TRUE) -> ()  [unwired: 1 in, 1 out]
          }
          frame #1 {
            n267 = call "Wait"("Count(Ticks)"=u32 20 ("Count(uSec)")) -> ()  [unwired: 1 out]
          }
          frame #2 {
            n268 = xnode "FPGA I/O Node"("PXI_Trig1"=FALSE) -> ()  [unwired: 1 in, 1 out]
          }
        }
      }
    }
  }
  n269 = node-c288() -> (w7:T4)  [unwired: 1 in]
  n270 = timed-loop "Trigger In Loop" {
    timing: w7 -> [_]
    timing-out: [_] -> w6
    stop <- FALSE stop-if-true
    # "Triggering is handeled in the 40MHz Loop to remove the signal Jitter and false triggers"
    n271 = xnode "FPGA I/O Node"() -> ("IO Module\\Asynchronous Trigger Input"=w561:bool)  [unwired: 1 in, 1 out]
    n272 = call <instrlib>:"Detect Rising Edge.vi"("signal"=w561) -> ("edge detected"=w558:bool)  [unwired: 14 in]
    n273 = xnode ("FIFO Method Node")("Element"=w561, "Timeout"=0) -> ()  [unwired: 1 in, 2 out]
    n274 = call-poly <instrlib>:"Count Up.vi"("increment"=w558, "reset"="Clear Count") -> ("count out"=→"Trig Count":u64)  [unwired: 13 in]
  }
  n275 = node-c288(w2) -> ()
  n276 = node-c288(w6) -> ()
  n277 = node-c288(w11) -> ()
